vi "Main_16a.vi"() -> ()   [LabVIEW 2023]
uses:
  ENUM_Type.ctl
  Cluster_Tracking point.ctl
  Cluster_Point.ctl
  ENUM_Direction_a2.ctl
  Map_Direction Next.ctl
panel:
  out "Answer 2":i32
  out "Array 2":cluster{"Track Point":T1[]}[](array[cluster])
  out "?":T4[][](array[typedef])
  in  "Puzzle":string="\\.......................|..-.............../../.......|...............\\.\\.....|..../.............|............\n........................../....../..............................-............-.-..--.........-...........\\/...\n....\\............../...........-...-......|.............................\\...............-........-....|.......\n......\\....|................./.\\................/..................../.......................|..\\......-......\n.................../..................-./.................../.....-...................|......\\.......|\\...\\./.\n.....|........../....................\\../..\\.../.\\.......-.............\\...........\\......|.\\..-..........-...\n..../............/.....\\...................../..--\\........|......\\....-...|.-...../......-........../........\n..............\\.-............./........./....|\\.......\\..........|.................|.|.................-......\n.....|..........-................-.../..........-........................\\.......|.........................-..\n.|.-......./....................\\........-.............../..\\.|.-\\...........\\./.................-............\n................|/............................../..-.\\..................-..../../...../.../..../..........|...\n........................./.....................\\..\\....-....../-.....................\\|.........././.-........\n...\\.....................-...../|............--......-..|...../.....|......|.../.\\....|.............\\|.......\\\n.........-...-.....|.........../...-/........|......./|............-.......-.....\\.............\\|....../......\n.....|...|.................|...../.............|.................../..........\\|..\\......|..|....-............\n...........................-.........\\......\\.............\\...................-.....-.\\.......-.....|.........\n.................-.............-......./.............-..\\./......|....-..-..........-....-............\\.......\n.\\..\\.......-......|........................\\.............-.......................|.........|\\.|..\\......--/..\n..........-.....||--........|........-....../...........|../...-.........../.....-.\\..........|.......-.......\n..........\\..........|..................\\.................-..../............/..........|.......-........../...\n..--......../..........-..|........./.........-...../........-.................|..\\............../.....-......\n.....\\.............|...../......../............./||..........................\\............|...................\n..-.................-|..-....................\\.................|...\\.....\\............./......-.......\\.......\n............-../......\\...../.-....-.....-....-./../......\\..|..|............................|.../..|.........\n-................./................................................|...............|....|.....-.....|....../..\n...........-...................|...........\\.......-..\\.......-...........|..-....../........|...............|\n.........|...|-........../...-..........|.........\\.....||......./....|...............\\......-......\\...../...\n....|.........|............\\.-.......................................-.......................|.-..|.\\...\\.-...\n.|....|....-/....................\\\\..........................|........\\|...|..............\\..|......-.\\../....\n..|.\\......|..../.....|.......-....................|.\\..\\............/......................|.....\\../../.....\n.......|\\\\.\\/......................./.............|................../.........|.....\\-.......................\n......................................../.../................\\-..............-................./......\\.......\n............../............/\\......./........................./......|............\\/..........................\n......./................|......../.........-............\\.../.|....../....|...../..../......../...............\n...................|............-\\........../...\\.......\\....\\.....-.........-./....|.........................\n.....-..-\\.................|\\...........................|..........\\........-...|.............................\n..............................-.............-.......\\......................../.......\\|.......|...-....-......\n\\...................\\..../.................\\................|......-...-............./.-......................\n........................./.|./...|..\\.-............|.-.....-..........\\....-..../.....|.......|...............\n.................../......../..................|.|...............|.......|\\.....|......|...............\\/..|..\n.........|....-......../........-./..|.../..|./...................-........|..................................\n..|../............-......-.........................-..|....-................-..\\....../...........|...........\n....................-...............|.../.....|..../......../...|.......\\.....-.....\\..............-..\\.-.....\n...........\\.........../............................................\\......-................-.......|.....-...\n..-............./.......-\\...........|-..-../............../................................../...............\n.................\\.......\\............../.|.......-...\\............................................\\.-........\n.\\....|....\\......|........./.....--......................................|................\\..|-..............\n......../...............-..........................|...........................-.............-\\.-..|..........\n.......|......|/...\\........./......../.....\\.........\\.......................-...........\\..\\................\n.-..-../.............|................./../.................\\........-......|.\\.....||...................\\|...\n/......../....\\.....|-..........\\..............-.....|............/\\......\\...//....................\\...-/....\n................-...........-.-\\-..........\\.-./......../-................./../.\\........................./...\n-.........-.....|.....-..|..|.........|...................-..........\\/.-.....................................\n......./...../......\\............-.|...............|..../.........|....\\.................../..............|...\n...........|.......|....|...............\\........................\\/..\\......................................\\.\n......\\........-.........................\\..........\\.............\\......................\\/.....\\..|..........\n......\\...........|.........../..-............./........................../...-......../...............\\..|...\n..|............\\../........../............\\...|.......................-...............\\-../.|...|\\.....\\......\n.|....\\.|....-|.........\\......./.................../.|........|....../.--.\\.....\\..............-\\\\.........-.\n......................./.......\\...........|.\\............-.....\\.............\\.........--......../.\\..-.|../.\n......../.............../......\\.\\....|.............../...........................-........-......../.........\n.......|\\.............|.../|/........../....\\.....-....|.............-......./........\\..\\........\\..|......-.\n.............../...........-.....\\..\\....-...../...|......\\...........................\\...|...........|/......\n.............|....../.................../..|.....................|.......|....//..............\\...............\n......./....\\............................-.........................-/......../|......-....|.............../...\n...........................|...................\\...............................-.................|...........\\\n.............................-......./..../...................\\.../...........-.|......................||.....\n\\....\\....\\...-./......../.........\\................./................\\...................|...........-.......\n................-.../............/\\..................\\.\\..-....../................./..........|...............\n......../...\\.......................\\.......\\..\\......|.....|../..........\\..........-.............|..........\n../.........................................-\\..........-.........|-./.....-...|..|.......\\........-...../../.\n.....|..........-......../|-..............|.................-...........|...\\.....................\\...........\n.......|..............\\....\\.....-............../..\\\\..\\.......-........./.........-..|...|................../\n..........-.......-.-................../.........\\\\...../.....|..........\\......./.|.............-...........\\\n..................................-..................|...........\\../\\...../..../...\\................/........\n...-.........................................................\\.|..............\\..................\\............\n-.|..|...................../../.|.......\\.....|.....\\.\\...\\.........-.................................../.....\n...\\./....../........\\.......-.................\\.........|............-.........../...........\\.|.........|.\\.\n..........-...\\.............-.-............-.-................/.....................|........|............-...\n|......./............/..|..............\\...............|.......|\\................/....|.........|.........\\..\\\n.....\\../\\./.....................-.............\\..................|.|.........................................\n............/......../.../.......\\............/.........................\\........................\\............\n....../..|.............../....................-.......\\................................................|.....\\\n................................../.......././.......\\.....|.\\......-.........-..||......../........-.//......\n........................\\.......|............-....-...../..............................-............-....|...-\n.....-.......|......\\..|.........-....|......\\......../..../.......\\..........|....\\.............||..\\........\n..........|...........-|.......\\.......-....../...../..........||.......................\\............-..|.....\n.................../../..............................|....|................/........|-....|................/..\n.....................\\................/............................/-........./...|.............\\...|..|\\.....\n.....\\..\\..........\\......../......|.........-....-..-..|...........\\....|./....\\.\\..\\............../.........\n.......-...............-....../...........-.......................|../...............|...|.........../..../...\n.............|.../..................\\..\\..........-........||................\\/...........-|..................\n.............-..............-\\.../.................|......\\...../..........\\...-.....-....../................\\\n.....-....................................-.........\\/............../.............................|...........\n./.|../......\\\\..........................................|..............\\|/..-\\..........................\\....\n...........-.........\\............./....-........-....-....-.........\\..\\....-\\...-...............--.........-\n..\\.............................\\............................./\\..........-.............-...-./........../....\n.................../........\\....|..-....|||./..............-......-./....................../..|...|..........\n......\\.........../............|\\...|.-................../....................|\\..|..\\.............-./......|.\n...........-...................-.|........................\\...............|/..-...\\...|/\\...........|.........\n............|..../..................................\\.......................\\........................-........\n.\\..........................|......|......../.|....................../.......\\......\\.............../.........\n..........-.../............/..........................|....-......................|.-................|.-......\n......../............-...|.....|......../-.....-|...|./.......-..................-\\...........................\n...............\\.\\/.-....././................-.../..../.............../-|.....-.......|......./..--...........\n..........-\\\\.|-................./../..|.-.....--................../.................../.|.......-............\n..\\.................-..............-...............\\.....|......................./..\\.....--........./..../..\\\n.......-....../..............|..................\\....|..|..........-.....|.|.-.........................\\......\n..../..\\...\\....................................||.|......................................|.......\\/.........-\n................\\-.-.....||....\\.........................-...................................................|"
  in  "Example":string=".|...\\....\n|.-.\\.....\n.....|-...\n........|.\n..........\n.........\\\n..../.\\\\..\n.-.-/..|..\n.|....-|.\\\n..//.|...."
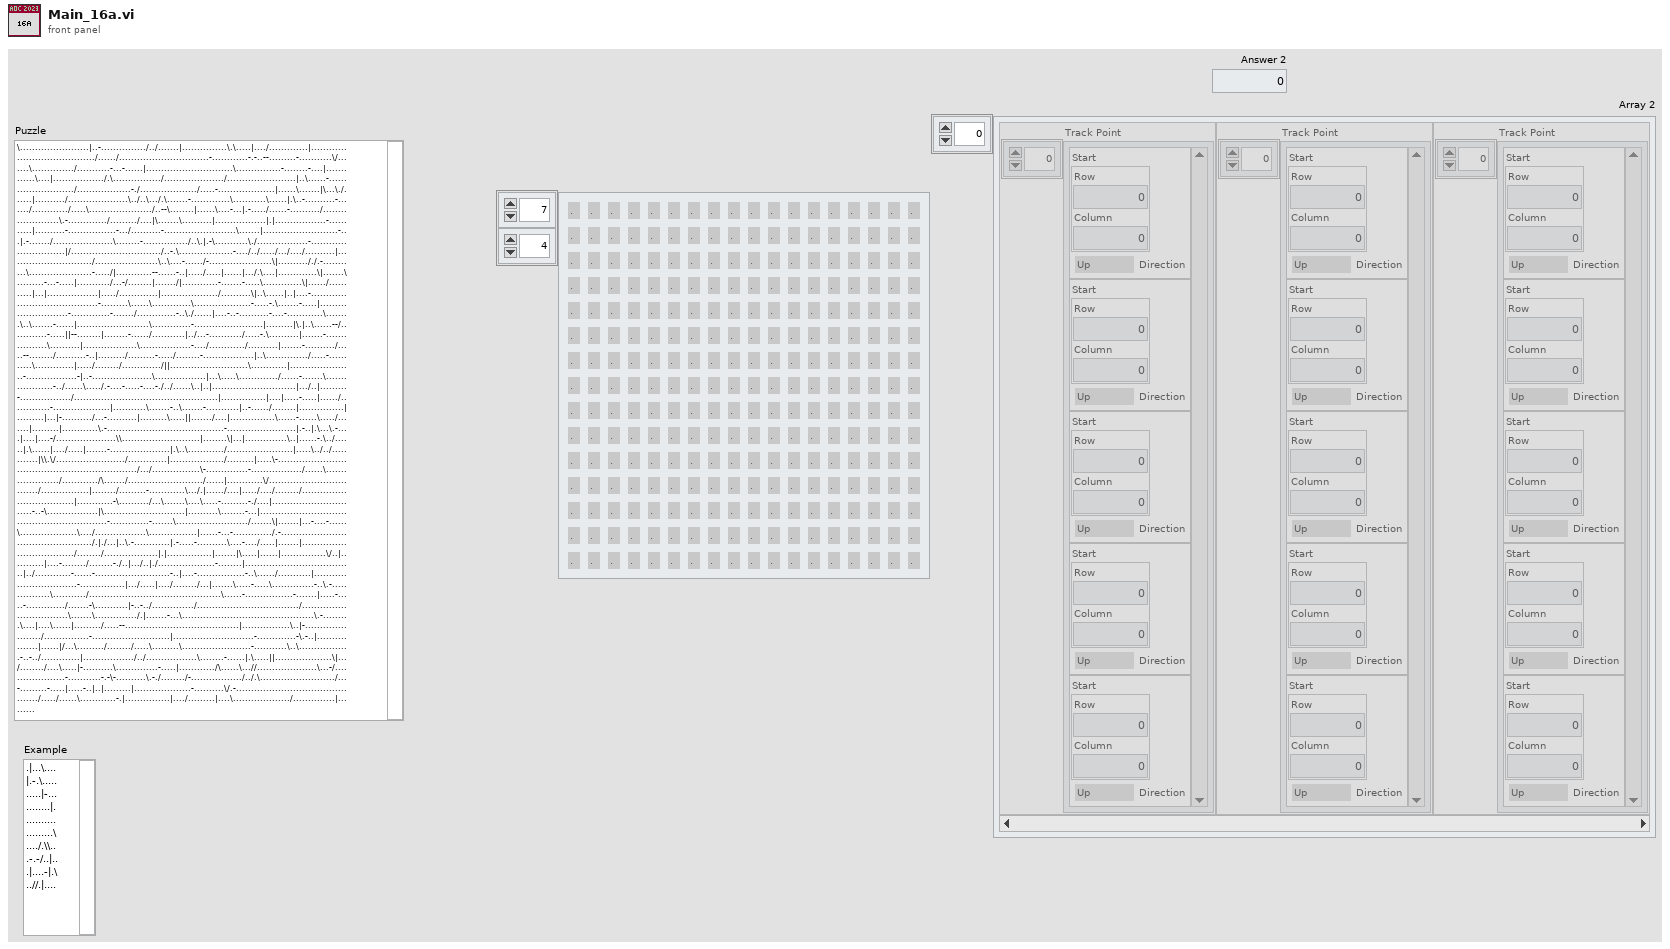
[diagram p1: front panel]
types:
  T1 = typedef "Cluster_Tracking point.ctl" = cluster{"Start":T2, "Direction":T3}
  T2 = typedef "Cluster_Point.ctl" = cluster{"Row":i32, "Column":i32}
  T3 = typedef "ENUM_Direction_a2.ctl" = enum16{"Up", "Left", "Down", "Right", "Up-Down", "Left-Right"}
  T4 = typedef "ENUM_Type.ctl" = enum16{".", "\\", "/", "|", "-"}
  T5 = typedef "Map_Direction Next.ctl" = map{T2, T3[]}
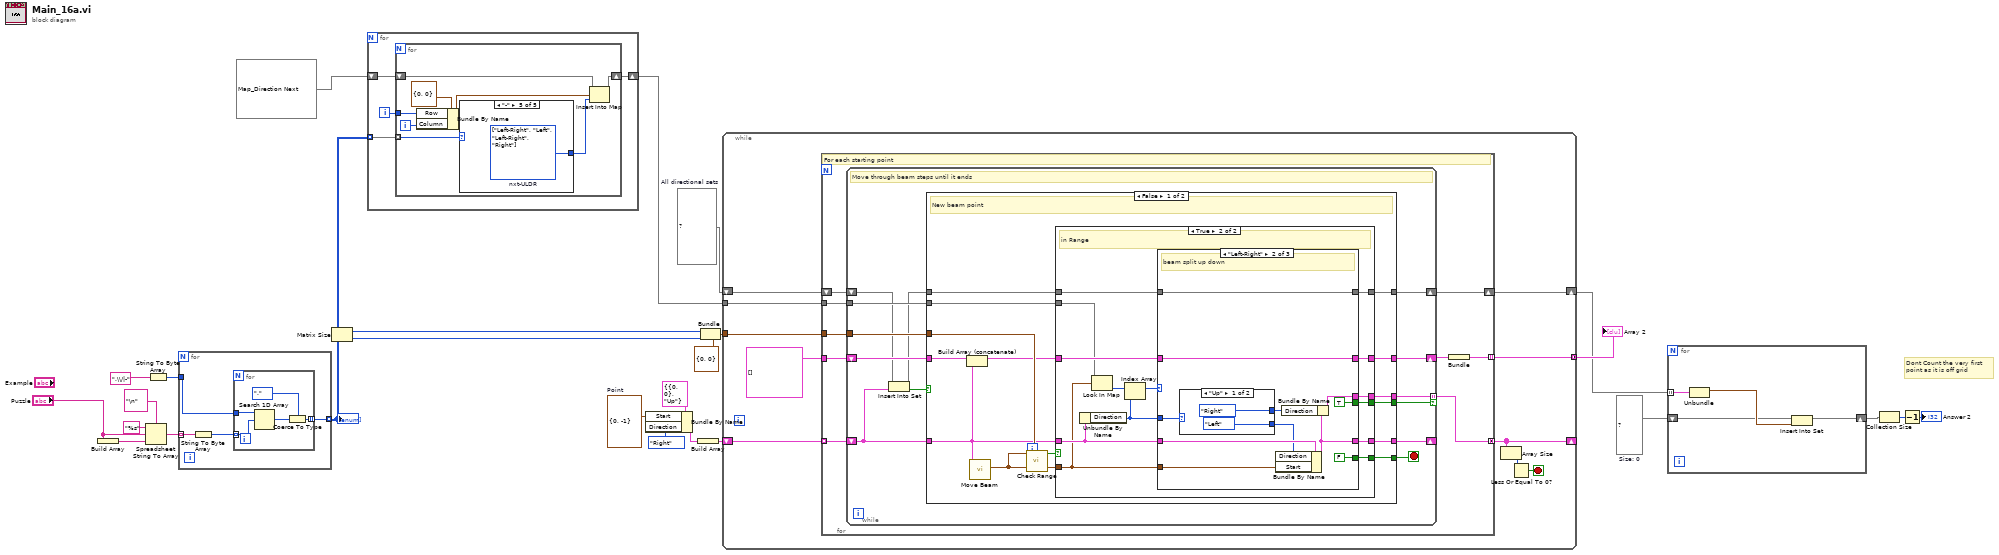
[diagram p0: block diagram]
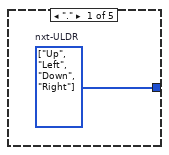
[diagram p2: hidden frame]
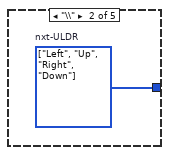
[diagram p3: hidden frame]
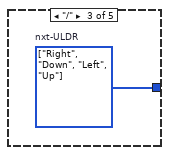
[diagram p4: hidden frame]
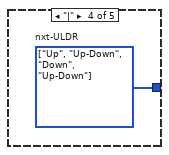
[diagram p5: hidden frame]
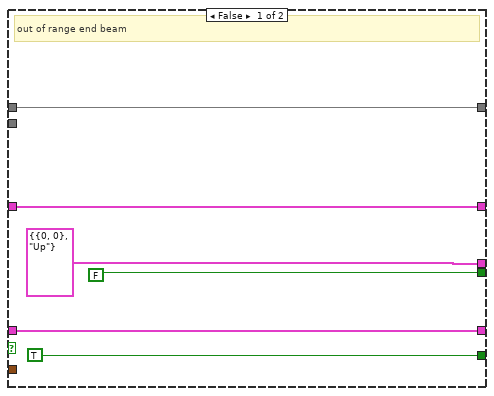
[diagram p6: hidden frame]
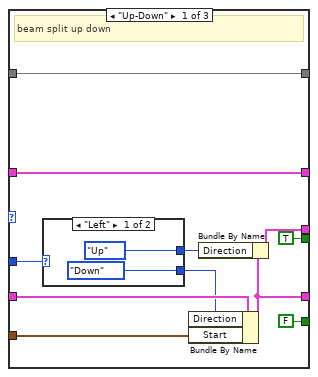
[diagram p7: hidden frame]
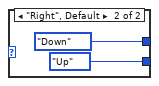
[diagram p8: hidden frame]
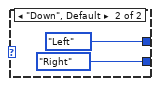
[diagram p9: hidden frame]
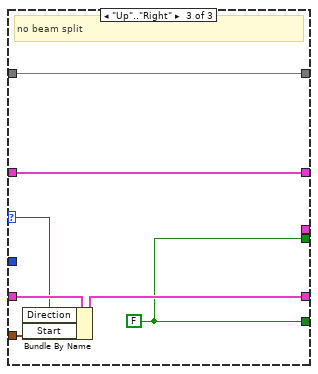
[diagram p10: hidden frame]
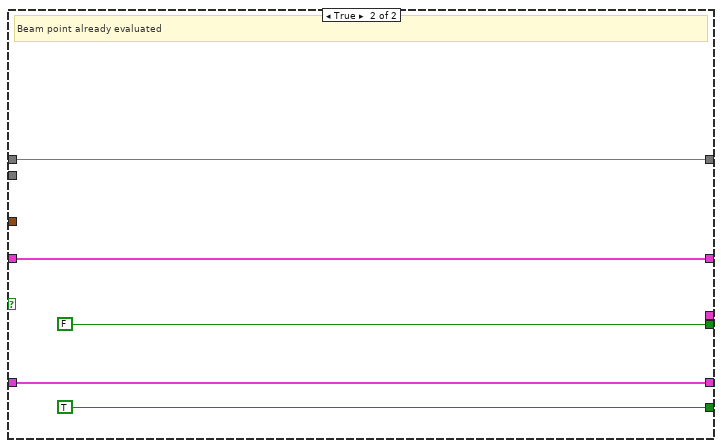
[diagram p11: hidden frame]
diagram:
  w6 = set{T2} {}  # Size: 0
  w8 = set{T1} {}  # All directional sets
  w19 = T2 {"Row"=0, "Column"=-1}  # Point
  # "Dont Count the very first\npoint as it is off grid"
  n1 = Build Array("Puzzle") -> (w26:string[])
  n2 = Spreadsheet String To Array(delimiter (Tab)="\n", format string="%s", spreadsheet string="Puzzle", array type (2D Dbl)=w26) -> (array=w23:string[])
  n3 = String To Byte Array(string=".\\/|-") -> (unsigned byte array=w21:u8[])
  n4 = for {
    tunnel: w23 -> [w30] mode=indexing
    tunnel: w21 -> [w29]
    tunnel: [w27] -> w16 mode=indexing
    n5 = String To Byte Array(string=w30) -> (unsigned byte array=w28:u8[])
    n6 = for {
      tunnel: w29 -> [w35]
      tunnel: w28 -> [w34] mode=indexing
      tunnel: [w31] -> w27 mode=indexing
      n7 = Search 1D Array(1D array=w35, element=w34) -> (index of element=w33:i32)  [unwired: 1 in]
      n8 = Coerce To Type(0:w33, 1:ENUM_Type."." ("Enum")) -> (2:w31:T4)
    }
  }
  "?" <- w16
  n9 = Matrix Size(0:w16) -> (1:w12:i32, 2:w11:i32)
  n10 = for {
    tunnel: w16 -> [w39] mode=indexing
    shift-right: [w36] -> w13
    shift-left: T5 {} -> [w37]
    i -> [w38]
    n11 = for {
      tunnel: w39 -> [w47] mode=indexing
      tunnel: w38 -> [w45]
      shift-right: [w42] -> w36
      shift-left: w37 -> [w43]
      i -> [w44]
      n12 = Bundle By Name(cluster=T2 {"Row"=0, "Column"=0} ("Start"), "Row"=w45, "Column"=w44) -> (w41:T2)
      n13 = case shown="\"-\"" w47 {
        tunnel: [w48 w49 w50 w51 w52] -> w40
        frame "." {
          w48 = T3[] [enum."Up", enum."Left", enum."Down", enum."Right"] items=["Up", "Left", "Down", "Right", "Up-Down", "Left-Right"]  # nxt-ULDR
        }
        frame "\\" {
          w49 = T3[] [enum."Left", enum."Up", enum."Right", enum."Down"] items=["Up", "Left", "Down", "Right", "Up-Down", "Left-Right"]  # nxt-ULDR
        }
        frame "/" {
          w50 = T3[] [enum."Right", enum."Down", enum."Left", enum."Up"] items=["Up", "Left", "Down", "Right", "Up-Down", "Left-Right"]  # nxt-ULDR
        }
        frame "|" {
          w51 = T3[] [enum."Up", enum."Up-Down", enum."Down", enum."Up-Down"] items=["Up", "Left", "Down", "Right", "Up-Down", "Left-Right"]  # nxt-ULDR
        }
        frame "-" {
          w52 = T3[] [enum."Left-Right", enum."Left", enum."Left-Right", enum."Right"] items=["Up", "Left", "Down", "Right", "Up-Down", "Left-Right"]  # nxt-ULDR
        }
      }
      n14 = Insert Into Map(map in=w43, key=w41, value=w40) -> (map out=w42:T5)  [unwired: 2 out]
    }
  }
  n15 = Bundle By Name(cluster=T1 {"Start"={"Row"=0, "Column"=0}, "Direction"=enum."Up"} ("Track Point"), "Start"=w19, "Direction"=ENUM_Direction_a2."Right") -> (w17:T1)
  n16 = Build Array(w17) -> (w20:T1[])
  n17 = Bundle(cluster=T2 {"Row"=0, "Column"=0} ("Point"), "Row"=w12, "Column"=w11) -> (w10:T2)
  n18 = while {
    tunnel: w13 -> [w62]
    shift-right: [w55] -> _
    shift-left: w20 -> [w60]
    shift-right: [w59] -> w3
    shift-left: w8 -> [w61]
    tunnel: w10 -> [w56]
    tunnel: [w53] -> w7 mode=concatenating
    stop <- w57 stop-if-true
    n19 = for {
      tunnel: w62 -> [w70]
      shift-right: [w71] -> w59
      shift-left: w61 -> [w67]
      tunnel: w60 -> [w66] mode=indexing
      tunnel: T1[] [] ("Track Point") -> [w68]
      tunnel: w56 -> [w69]
      tunnel: [w65] -> w55 mode=concatenating
      tunnel: [w63] -> w53 mode=indexing
      # "For each starting point"
      n20 = while {
        tunnel: w70 -> [w83]
        tunnel: w69 -> [w82]
        shift-right: [w84] -> w71
        shift-left: w67 -> [w74]
        shift-right: [w79] -> w64
        shift-left: w68 -> [w81]
        shift-right: [w76] -> _
        shift-left: w66 -> [w75]
        tunnel: [w78] -> w65 mode=indexing if=w77
        stop <- w80 stop-if-true
        # "Move through beam steps until it ends"
        n21 = Insert Into Set(10:w75, 11:w74) -> (2:w72:bool, 3:w73:set{T1})
        n22 = case shown="False" w72 {
          tunnel: [w98 w160] -> w84
          tunnel: w83 -> [w97 _]
          tunnel: w82 -> [w96 _]
          tunnel: w81 -> [w87 w156]
          tunnel: [w93 TRUE] -> w80
          tunnel: [w92 w156] -> w79
          tunnel: [w91 _] -> w78
          tunnel: [w90 FALSE] -> w77
          tunnel: [w89 w158] -> w76
          tunnel: w75 -> [w85 w158]
          tunnel: w73 -> [w88 w160]
          frame False {
            # "New beam point"
            n23 = Build Array (concatenate)(w87, w85) -> (w86:T1[])
            n24 = call "Move Beam.vi"("Track Point"=w85) -> ("Next Position Out"=w95:T2)  [unwired: 9 in, 1 out]
            n25 = call "Check Range.vi"("Range"=w96, "Next Position"=w95) -> ("In Range Out"=w94:bool)  [unwired: 9 in]
            n26 = case shown="True" w94 {
              tunnel: [w103 w118] -> w98
              tunnel: w85 -> [w99 w111]
              tunnel: w88 -> [w103 w117]
              tunnel: w86 -> [w100 w116]
              tunnel: w95 -> [_ w109]
              tunnel: w97 -> [_ w113]
              tunnel: [TRUE w108] -> w93
              tunnel: [w100 w114] -> w92
              tunnel: [T1 {"Start"={"Row"=0, "Column"=0}, "Direction"=enum."Up"} ("Track Point") w105] -> w91
              tunnel: [FALSE w107] -> w90
              tunnel: [w99 w115] -> w89
              frame False {
                # "out of range end beam"
              }
              frame True {
                # "in Range"
                n27 = Unbundle By Name(w111) -> ("Direction"=w106:T3)
                n28 = Look In Map(map=w113, key=w109) -> (value=w112:T3[])  [unwired: 1 in, 1 out]
                n29 = Index Array(array=w112, index=w106) -> (element=w110:T3)
                n30 = case shown="\"Left-Right\"" w110 {
                  selector: w110 -> [_ _ w149]
                  tunnel: w116 -> [w127 w142 w155]
                  tunnel: [w127 w142 w155] -> w114
                  tunnel: w117 -> [w128 w143 w154]
                  tunnel: [w128 w143 w154] -> w118
                  tunnel: w111 -> [w129 w144 w152]
                  tunnel: [w120 w135 w153] -> w115
                  tunnel: w109 -> [w123 w138 w151]
                  tunnel: [FALSE FALSE w150] -> w108
                  tunnel: [TRUE TRUE w150] -> w107
                  tunnel: w106 -> [w126 w141 _]
                  tunnel: [w122 w137 _] -> w105
                  frame "Up-Down" {
                    # "beam split up down"
                    n31 = case shown="\"Left\"" w126 {
                      tunnel: [ENUM_Direction_a2."Down" ("Direction") ENUM_Direction_a2."Up" ("Direction")] -> w125
                      tunnel: [ENUM_Direction_a2."Up" ("Direction") ENUM_Direction_a2."Down" ("Direction")] -> w124
                      frame "Left" {
                      }
                      frame "Right", Default {
                      }
                    }
                    n32 = Bundle By Name(cluster=w129, "Direction"=w125, "Start"=w123) -> (w120:T1)
                    n33 = Bundle By Name(cluster=w120, "Direction"=w124) -> (w122:T1)
                  }
                  frame "Left-Right" {
                    # "beam split up down"
                    n34 = case shown="\"Up\"" w141 {
                      tunnel: [ENUM_Direction_a2."Left" ("Direction") ENUM_Direction_a2."Right" ("Direction")] -> w140
                      tunnel: [ENUM_Direction_a2."Right" ("Direction") ENUM_Direction_a2."Left" ("Direction")] -> w139
                      frame "Up" {
                      }
                      frame "Down", Default {
                      }
                    }
                    n35 = Bundle By Name(cluster=w144, "Direction"=w140, "Start"=w138) -> (w135:T1)
                    n36 = Bundle By Name(cluster=w135, "Direction"=w139) -> (w137:T1)
                  }
                  frame "Up".."Right" {
                    w150 = FALSE
                    # "no beam split"
                    n37 = Bundle By Name(cluster=w152, "Direction"=w149, "Start"=w151) -> (w153:T1)
                  }
                }
              }
            }
          }
          frame True {
            # "Beam point already evaluated"
          }
        }
      }
      n38 = Bundle("Track Point"=w64) -> (w63:cluster{"Track Point":T1[]})  [unwired: 1 in]
    }
    n39 = Array Size(array=w55) -> (size(s)=w58:i32)
    n40 = Less Or Equal To 0?(x=w58) -> (x <= 0?=w57:bool)
  }
  "Array 2" <- w7
  n41 = for {
    tunnel: w3 -> [w164] mode=indexing
    shift-right: [w161] -> w5
    shift-left: w6 -> [w162]
    n42 = Unbundle(w164) -> ("Start"=w163:T2)  [unwired: 1 out]
    n43 = Insert Into Set(10:w163, 11:w162) -> (3:w161:set{T2})  [unwired: 1 out]
  }
  n44 = Collection Size(1:w5) -> (0:w4:i32)
  n45 = Decrement(x=w4) -> (x-1=→"Answer 2":i32)
